vi "Get stack data.vi"(8 "error in (no error)":errorcluster, 11 "Stack in":refnum<class "Stack.lvclass">) -> (0 "error out":errorcluster, 1 "Is real run":bool, 2 "Data cluster":T1={"type (proto/module)"="proto", " geometry"="full", "resolution"="LD", "baselayer"="BA_123", "toplayer"="SI_789", "bl_pos"="1", "tl_pos"="1", "put_pos"="1", "region"="1", "asstray"="1", "comptray"="1", "put"="1", "date"="2024-04-02", "timestart"="1:12:12.442", "timeend"="1:23:45.244", "operator"="cmuperson", "tape"="some", "glue"="some", "stack name"="some", "Adhesive type"="", "Comments"="", "Temperature"="", "Relative Humidity"=""}, 3 "Stack out":refnum<class "Stack.lvclass">)   [LabVIEW 2021, in "Stack.lvclass"]
uses:
  Stack.lvclass
  Stack.lvclass/Stack.ctl
panel:
  # "Debug Instructions\n#### The order of values in db_data_cols must match the order of values in Data cluster in Stack.lvclass: Get stack data.vi \n#### The variable names below correspond to postgres col name. LV does not neet to match the col numes but just the values. \n#### Right-click on the Data cluster on the front panel and click on 'reorder controls' to verify the order is correct in the code. \n#### The physical position of the fields is different from the actual position.\n\nIn Main VIs/python_db/postgres_tools.py, see functions 'assembly_data' and 'assembly_data_as_list'."
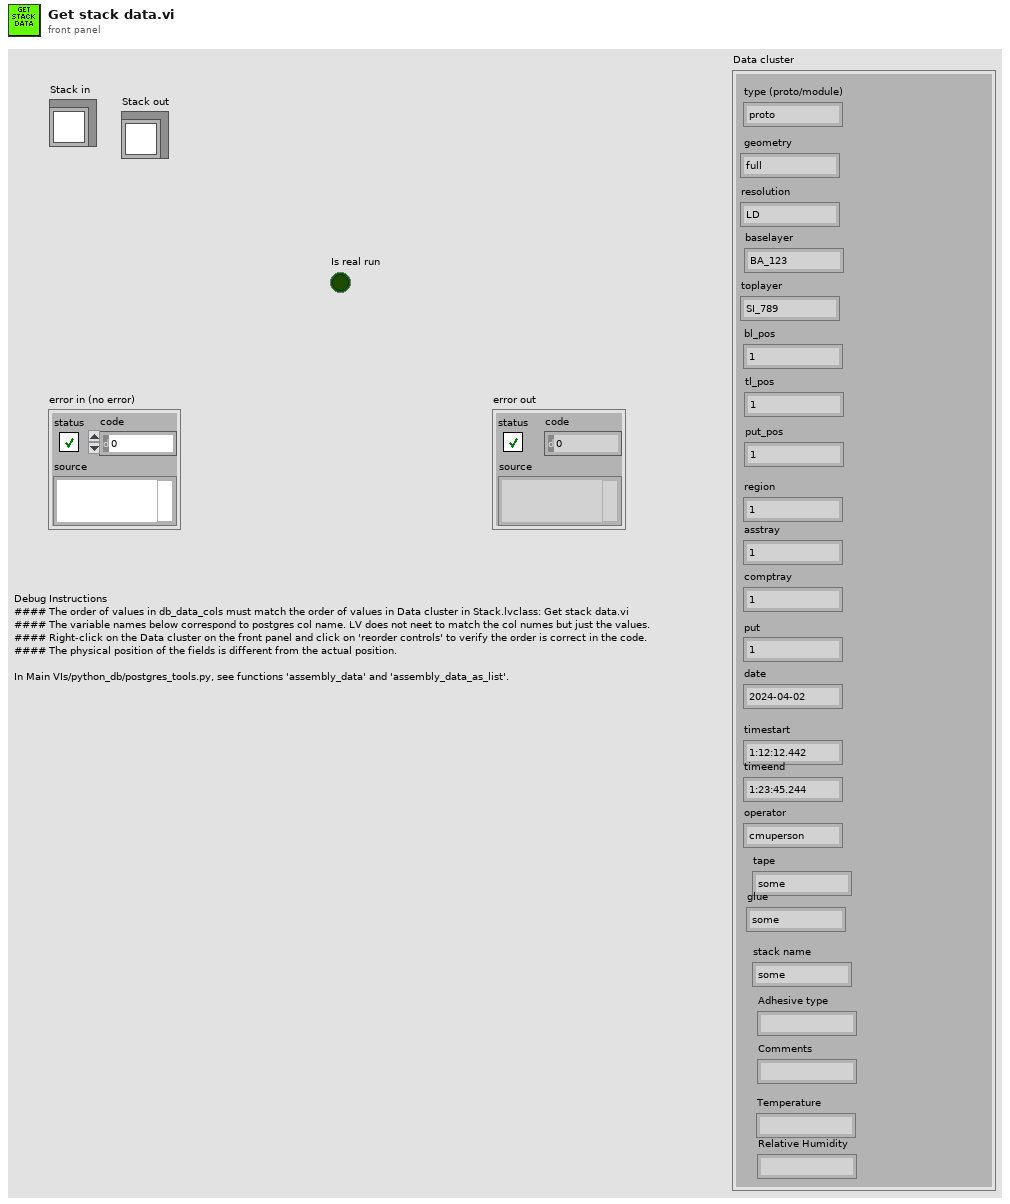
[diagram p1: front panel]
types:
  T1 = cluster{"type (proto/module)":string, " geometry":string, "resolution":string, "baselayer":string, "toplayer":string, "bl_pos":string, "tl_pos":string, "put_pos":string, "region":string, "asstray":string, "comptray":string, "put":string, "date":string, "timestart":string, "timeend":string, "operator":string, "tape":string, "glue":string, "stack name":string, "Adhesive type":string, "Comments":string, "Temperature":string, "Relative Humidity":string}
  T2 = cluster{"type":string, " geometry":string, "resolution":string, "baselayer":string, "toplayer":string, "bl_pos":string, "tl_pos":string, "put_pos":string, "region":string, "asstray":string, "comptray":string, "put":string, "date":string, "timestart":string, "timeend":string, "operator":string, "tape":string, "glue":string, "stack name":string, "Adhesive type":string, "Comments":string, "Temperature":string, "Relative Humidity":string}
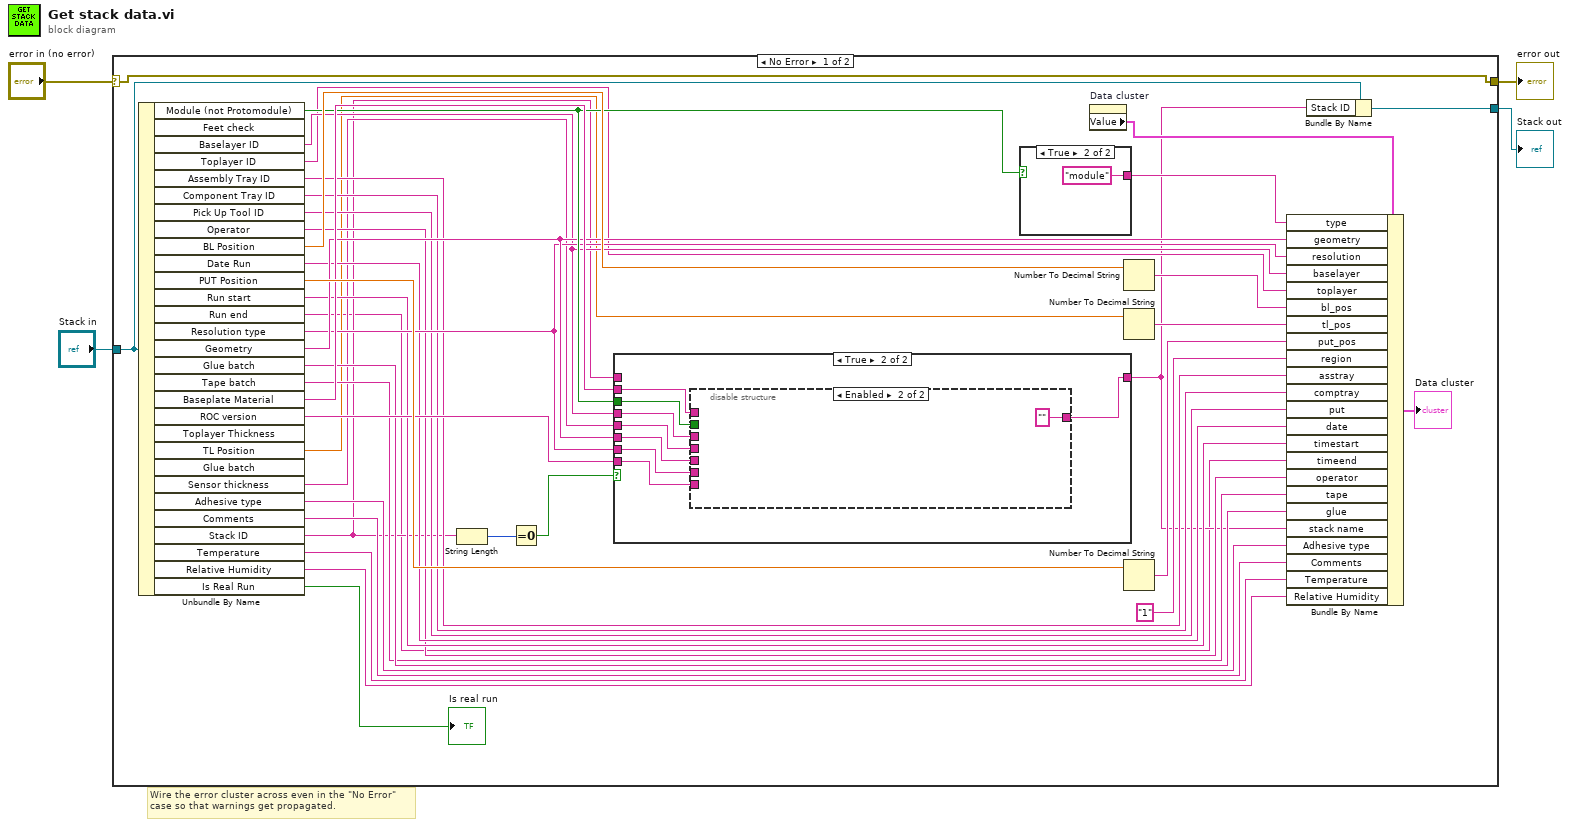
[diagram p0: block diagram]
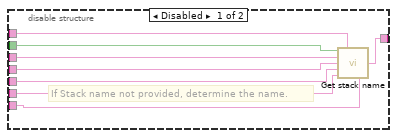
[diagram p3: hidden frame]
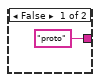
[diagram p4: hidden frame]
diagram:
  # "Wire the error cluster across even in the \"No Error\"\ncase so that warnings get propagated."
  n1 = case shown="No Error" "error in (no error)" {
    selector: "error in (no error)" -> [w43 w65]
    tunnel: [w43 w65] -> w3
    tunnel: [w9 w64] -> w1
    tunnel: "Stack in" -> [w8 w64]
    frame No Error {
      n2 = Unbundle By Name(w8) -> ("Module (not Protomodule)"=w39:bool, "Baselayer ID"=w32:string, "Toplayer ID"=w31:string, "Assembly Tray ID"=w30:string, "Component Tray ID"=w29:string, "Pick Up Tool ID"=w28:string, "Operator"=w25:string, "BL Position"=w42:dbl, "Date Run"=w27:string, "PUT Position"=w41:dbl, "Run start"=w26:string, "Run end"=w6:string, "Resolution type"=w33:string, "Geometry"=w34:string, "Glue batch"=w24:string, "Tape batch"=w23:string, "Baseplate Material"=w40:string, "ROC version"=w38:string, "TL Position"=w22:dbl, "Sensor thickness"=w17:string, "Adhesive type"=w16:string, "Comments"=w15:string, "Stack ID"=w12:string, "Temperature"=w11:string, "Relative Humidity"=w10:string, "Is Real Run"=→"Is real run":bool)  [unwired: 3 out]
      n3 = String Length(string=w12) -> (length=w14:i32)
      n4 = Equal To 0?(x=w14) -> (x = 0?=w13:bool)
      n5 = case shown="True" w13 {
        tunnel: w40 -> [_ w52]
        tunnel: w39 -> [_ w51]
        tunnel: w38 -> [_ w50]
        tunnel: [w44 w49] -> w7
        tunnel: w34 -> [_ w48]
        tunnel: w33 -> [_ w47]
        tunnel: w32 -> [_ w46]
        tunnel: w17 -> [_ w45]
        tunnel: w12 -> [w44 _]
        frame False {
        }
        frame True {
          n6 = disable-structure shown="Enabled" {
            disable-tunnel: w52 -> [w60 _]
            disable-tunnel: w51 -> [w59 _]
            disable-tunnel: w50 -> [w58 _]
            disable-tunnel: [w57 "" ("Stack name")] -> w49
            disable-tunnel: w48 -> [w56 _]
            disable-tunnel: w47 -> [w55 _]
            disable-tunnel: w46 -> [w54 _]
            disable-tunnel: w45 -> [w53 _]
            frame Disabled {
              # "If Stack name not provided, determine the name."
              n7 = call "Get stack name.vi"("Module?"=w59, "Baseplate Type"=w60, "Protoname (baselayer)"=w54, "Sensor thickness"=w53, "Geometry"=w56, "Resolution"=w55, "Hexaboard ROC version"=w58) -> ("Stack name"=w57:string)  [unwired: 8 in]
            }
            frame Enabled {
            }
          }
        }
      }
      n8 = case shown="True" w39 {
        tunnel: ["proto" ("type") "module" ("type")] -> w35
        frame False {
        }
        frame True {
        }
      }
      n9 = property on="Data cluster" class="Clust (strict)"() -> ("Value"=w36:T2)  [unwired: 2 in, 2 out]
      n10 = Number To Decimal String(number=w42) -> (decimal integer string=w20:string)  [unwired: 1 in]
      n11 = Number To Decimal String(number=w22) -> (decimal integer string=w21:string)  [unwired: 1 in]
      n12 = Number To Decimal String(number=w41) -> (decimal integer string=w19:string)  [unwired: 1 in]
      n13 = Bundle By Name(cluster=w36, "type"=w35, "geometry"=w34, "resolution"=w33, "baselayer"=w32, "toplayer"=w31, "bl_pos"=w20, "tl_pos"=w21, "put_pos"=w19, "region"="1", "asstray"=w30, "comptray"=w29, "put"=w28, "date"=w27, "timestart"=w26, "timeend"=w6, "operator"=w25, "tape"=w23, "glue"=w24, "stack name"=w7, "Adhesive type"=w16, "Comments"=w15, "Temperature"=w11, "Relative Humidity"=w10) -> (→"Data cluster":T2)
      n14 = Bundle By Name(cluster=w8, "Stack ID"=w7) -> (w9:refnum<class "Stack.lvclass">)
    }
    frame Error {
    }
  }
  "error out" <- w3
  "Stack out" <- w1
